vi "Noise signal.vi"(8 "错误输入":errorcluster, 9 "写入（非为读取）":bool, 10 "input signal":dbl[](array[numeric]), 11 "Path":string) -> (0 "错误输出":errorcluster, 3 "output signal":dbl[](array[numeric]))   [LabVIEW 2015, in "Digital Signal Processing.lvlib"]
uses:
  Digital Signal Processing.lvlib
  <vilib>/Utility/file.llb/Read Delimited Spreadsheet (DBL).vi
  <vilib>/Utility/file.llb/Write Delimited Spreadsheet (DBL).vi
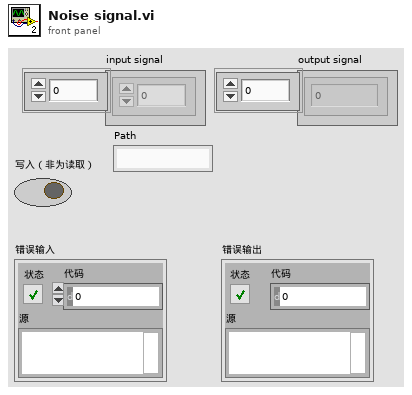
[diagram p1: front panel]
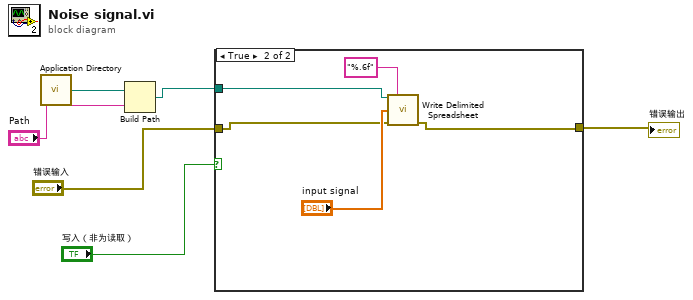
[diagram p0: block diagram]
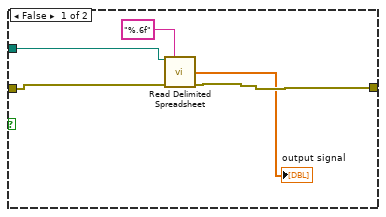
[diagram p2: hidden frame]
diagram:
  n1 = call <vilib>:"Application Directory.vi"() -> ("Application Directory"=w6:path)
  n2 = Build Path(base path=w6, name or relative path="Path") -> (appended path=w3:path)
  n3 = case shown="True" "写入（非为读取）" {
    tunnel: "错误输入" -> [w10 w14]
    tunnel: [w9 w13] -> w1
    tunnel: w3 -> [w11 w16]
    frame False {
      n4 = call-poly <vilib>:"Read Delimited Spreadsheet.vi"("file path (dialog if empty)"=w11, "format (%.3f)"="%.6f", "error in (no error)"=w10) -> ("first row"=→"output signal":dbl[], "error out"=w9:errorcluster)  [unwired: 7 in, 4 out]
    }
    frame True {
      n5 = call-poly <vilib>:"Write Delimited Spreadsheet.vi"("file path (dialog if empty)"=w16, "format (%.3f)"="%.6f", "1D data"="input signal", "error in (no error)"=w14) -> ("error out"=w13:errorcluster)  [unwired: 10 in, 1 out]
    }
  }
  "错误输出" <- w1
